vi "ExtractDownloadedBinaryBuilds.vi"   [LabVIEW 2020]
uses:
  <vilib>/Utility/sysdir.llb/System Directory Type.ctl
  <vilib>/zip/NI_Unzip.lvlib
types:
  T1 = typedef "System Directory Type.ctl" = i32
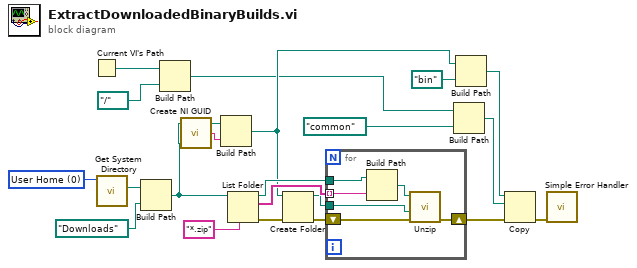
[diagram p0: block diagram]
diagram:
  w20 = T1 0 items=["User Home"=0, "User Desktop"=1, "User Documents"=2, "User Application Data"=3, "User Preferences"=4, "User Temporary"=5, "Public Documents"=6, "Public Application Data"=7, "Public Preferences"=8, "Public Cache"=13, "System Core Libraries"=9, "System Installed Libraries"=10, "Application Files"=11, "Boot Volume Root"=12] ("system directory type")
  n1 = Current VI's Path() -> (path=w2:path)
  n2 = call <vilib>:"Get System Directory.vi"("system directory type"=w20) -> ("system directory"=w21:path)  [unwired: 10 in]
  n3 = Build Path(base path=w21, name or relative path=path "Downloads") -> (appended path=w5:path)
  n4 = Build Path(base path=w2, name or relative path=path "../..") -> (appended path=w3:path)
  n5 = call <vilib>:"Create NI GUID.vi"() -> ("NI GUID"=w14:string)
  n6 = Build Path(base path=w5, name or relative path=w14) -> (appended path=w4:path)
  n7 = List Folder(path=w5, pattern="*.zip") -> (path out=w16:path, filenames=w17:string[], error out=w13:errorcluster)  [unwired: 2 in, 1 out]
  n8 = Create Folder(path (use dialog)=w4, error in=w13) -> (created path=w6:path, error out=w12:errorcluster)  [unwired: 1 in, 1 out]
  n9 = for {
    tunnel: w17 -> [w26] mode=indexing
    tunnel: w16 -> [w23]
    shift-right: [w24] -> w11
    shift-left: w12 -> [w27]
    tunnel: w6 -> [w22]
    n10 = Build Path(base path=w23, name or relative path=w26) -> (appended path=w25:path)
    n11 = call <vilib>:"Unzip.vi"("error in (no error)"=w27, "Target directory (same as Zip file if empty)"=w22, "Zip file"=w25) -> ("error out"=w24:errorcluster)  [unwired: 6 in, 2 out]
  }
  n12 = Build Path(base path=w3, name or relative path=path "common" ("Path")) -> (appended path=w9:path)
  n13 = Build Path(base path=w4, name or relative path=path "bin") -> (appended path=w8:path)
  n14 = Copy(8:w11, 10:w9, 11:w8) -> (0:w7:errorcluster)  [unwired: 2 in, 2 out]
  n15 = call <vilib>:"Simple Error Handler.vi"("error in (no error)"=w7) -> ()  [unwired: 4 in, 5 out]
